vi "Compare ISO8601 DateTimes.vi"(1 "Unit (ms)":T1=enum."millisecond", 2 "ISO8601 DateTime (1)":string, 3 "ISO8601 DateTime (2)":string, 4 "Resolution (in selected unit)":dbl=1.0) -> (7 "Equal?":bool)   [LabVIEW 2013]
doc: "Timestamp is not converted to UTC time, so the year being evaluated is the year of the timestamp, not the current year at GMT."
uses:
  Timestamp Compare Units -- enum.ctl
  EpochNotTimestamp.vi
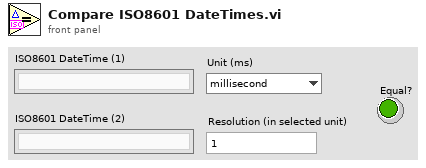
[diagram p1: front panel]
types:
  T1 = typedef "Timestamp Compare Units -- enum.ctl" = enum16{"week", "day", "hour", "minute", "second", "millisecond", "microsecond", "nanosecond"}
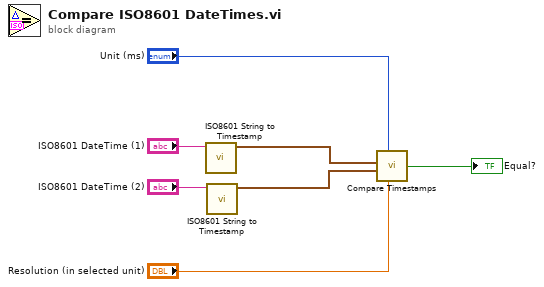
[diagram p0: block diagram]
diagram:
  n1 = call "ISO8601 String to Timestamp.vi"("ISO8601 String"="ISO8601 DateTime (1)") -> ("Timestamp"=w3:timestamp)  [unwired: 8 in, 2 out]
  n2 = call "ISO8601 String to Timestamp.vi"("ISO8601 String"="ISO8601 DateTime (2)") -> ("Timestamp"=w1:timestamp)  [unwired: 8 in, 2 out]
  n3 = call "Compare Timestamps.vi"("Unit (ms)"="Unit (ms)", "timestamp (1)"=w3, "timestamp (2)"=w1, "Resolution (in selected unit)"="Resolution (in selected unit)") -> ("Equal?"=→"Equal?":bool)  [unwired: 4 in]
